vi "getSerializedData.vi"(0 "reference in":refnum<class "VINode.lvclass">, 5 "error in (no error)":errorcluster) -> (14 "reference out":refnum<class "VINode.lvclass">, 15 "parent":refnum<class "AbstractNode.lvclass">, 16 "children":refnum<class "AbstractNode.lvclass">[](array[class]), 17 "xmlOut":string, 19 "error out":errorcluster)   [LabVIEW 2016, in "VINode.lvclass"]
doc: "Gets data to store"
uses:
  <resource>/Framework/Providers/Open_GDS/UML/VINode_class/VINode.lvclass
  C:/Program Files (x86)/National Instruments/LabVIEW 2016/resource/Framework/Providers/Open_GDS/UML/AbstractNode_class/AbstractNode.lvclass
  C:/Program Files (x86)/National Instruments/LabVIEW 2016/resource/Framework/Providers/Open_GDS/UML/RectangularNode_class/RectangularNode.lvclass
  <resource>/Framework/Providers/Open_GDS/UML/AbstractNode_class/AbstractNode.lvclass
  <resource>/Framework/Providers/Open_GDS/UML/MultiLineString_class/MultiLineString.lvclass
  <resource>/Framework/Providers/Open_GDS/UML/RectangularNode_class/RectangularNode.lvclass
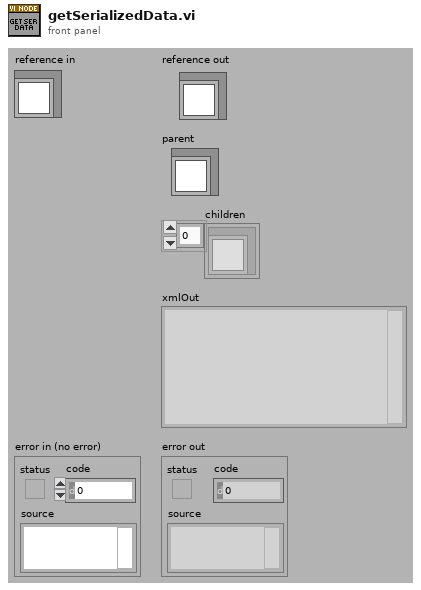
[diagram p1: front panel]
types:
  T1 = typedef "AbstractNode.lvclass/ObjectAttributes.ctl" = cluster{"parent":refnum<class "AbstractNode.lvclass">, "children":refnum<class "AbstractNode.lvclass">[], "Hidden":bool}
  T2 = typedef "RectangularNode.lvclass/ObjectAttributes.ctl" = cluster{"bounds":T3}
  T3 = typedef "Rectangle Rectangle2D.ctl" = cluster{"x":dbl, "y":dbl, "width":dbl, "height":dbl}
  T4 = typedef "VINode.lvclass/ObjectAttributes.ctl" = cluster{"midHeight":dbl, "botHeight":dbl, "Name":refnum<class "MultiLineString.lvclass">, "DEFAULT_COMPARTMENT_HEIGHT":i32, "DEFAULT_WIDTH":i32, "DEFAULT_HEIGHT":i32, "VIPath":path, "Description":refnum<class "MultiLineString.lvclass">, "ShowDescription":bool}
  T5 = cluster{"data string":string, "text":string, "text":string}
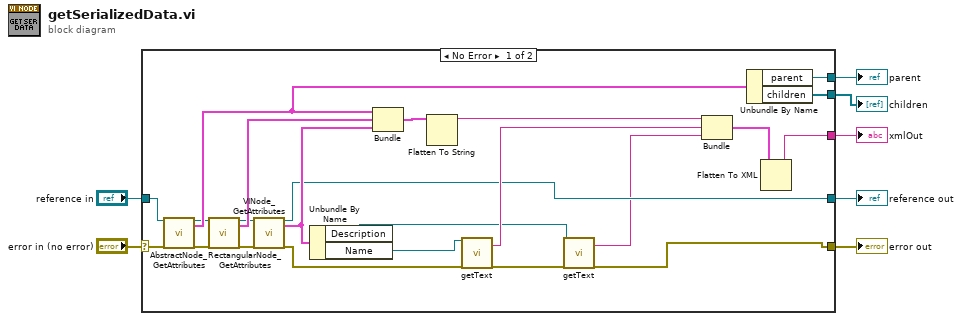
[diagram p0: block diagram]
diagram:
  n1 = case shown="No Error" "error in (no error)" {
    selector: "error in (no error)" -> [w19 w31]
    tunnel: "reference in" -> [w18 w32]
    tunnel: [w10 w31] -> w5
    tunnel: [w14 w32] -> w4
    tunnel: [w30 _] -> w3
    tunnel: [w29 _] -> w2
    tunnel: [w28 _] -> w1
    frame No Error {
      n2 = call <resource>:"AbstractNode_GetAttributes.vi"("reference in"=w18, "error in (no error)"=w19) -> ("reference out"=w16:refnum<class "VINode.lvclass">, "Data"=w24:T1, "error out"=w20:errorcluster)  [unwired: 14 in, 1 out]
      n3 = call <resource>:"RectangularNode_GetAttributes.vi"("reference in"=w16, "error in (no error)"=w20) -> ("reference out"=w17:refnum<class "VINode.lvclass">, "Data"=w23:T2, "error out"=w21:errorcluster)  [unwired: 14 in, 1 out]
      n4 = call <resource>:"VINode_GetAttributes.vi"("reference in"=w17, "error in (no error)"=w21) -> ("reference out"=w14:refnum<class "VINode.lvclass">, "Data"=w22:T4, "error out"=w15:errorcluster)  [unwired: 1 in, 14 out]
      n5 = Unbundle By Name(w22) -> ("Description"=w8:refnum<class "MultiLineString.lvclass">, "Name"=w25:refnum<class "MultiLineString.lvclass">)
      n6 = Bundle("Data"=w24, "Data"=w23, "Data"=w22) -> (w13:cluster{"Data":T1, "Data":T2, "Data":T4})  [unwired: 1 in]
      n7 = Flatten To String(anything=w13) -> (data string=w12:string)  [unwired: 3 in, 2 out]
      n8 = call-dynamic "getText.vi"("reference"=w25, "error in (no error)"=w15) -> ("text"=w26:string, "error out"=w11:errorcluster)  [unwired: 16 out]
      n9 = call-dynamic "getText.vi"("reference"=w8, "error in (no error)"=w11) -> ("text"=w9:string, "error out"=w10:errorcluster)  [unwired: 16 out]
      n10 = Bundle("data string"=w12, "text"=w26, "text"=w9) -> (w27:T5)  [unwired: 1 out]
      n11 = Unbundle By Name(w24) -> ("parent"=w30:refnum<class "AbstractNode.lvclass">, "children"=w29:refnum<class "AbstractNode.lvclass">[])
      n12 = Flatten To XML(anything=w27) -> (xml string=w28:string)
    }
    frame Error {
    }
  }
  "reference out" <- w4
  "error out" <- w5
  "children" <- w2
  "parent" <- w3
  "xmlOut" <- w1
